vi "BatchModeDeactivate.vi"(11 "client handle in":T1) -> (3 "client handle out":T1)   [LabVIEW 2020]
uses:
  <vilib>/httpClient/ClientHandle.ctl
  <vilib>/httpClient/LabVIEWHTTPClient.lvlib
  <vilib>/wsapi/NI_WebServices.lvlib
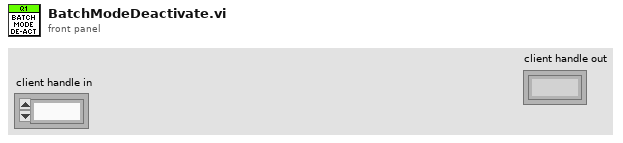
[diagram p1: front panel]
types:
  T1 = typedef "LabVIEWHTTPClient.lvlib/ClientHandle.ctl" = refnum<k1>
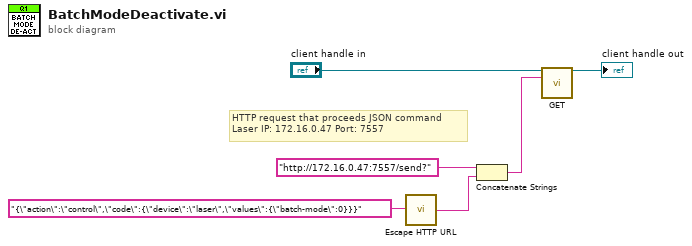
[diagram p0: block diagram]
diagram:
  # "HTTP request that proceeds JSON command\nLaser IP: 172.16.0.47 Port: 7557"
  n1 = call <vilib>:"Escape HTTP URL.vi"("unescaped string in"="{\"action\":\"control\",\"code\":{\"device\":\"laser\",\"values\":{\"batch-mode\":0}}}" ("JSON command")) -> ("escaped string out"=w6:string)
  n2 = Concatenate Strings("http://172.16.0.47:7557/send?", w6) -> (w5:string)
  n3 = call <vilib>:"GET.vi"("client handle"="client handle in", "url"=w5) -> ("client handle out"=→"client handle out":T1)  [unwired: 10 in, 3 out]
